vi "popUPCrearNuevoObjetoReceta.vi"() -> (2 "datosReceta":T1, 3 "Listo Ingresar OD SteelGrade Lote":bool=TRUE)   [LabVIEW 2014]
panel:
  in  "textoFinCarga":string="Gracias por ingresar los datos de la receta"
  in  "ingresarIDStadisctic":string="numeroIdStad"
  in  "ingresarDataCreate":string="camposMedicion"
  in  "ingresarIDReceta":string="numeroIDReceta"
  in  "ingresarCamposMedicion":string="numLote"
  in  "ingresarSteelGrade":string="numSteelGrade"
  in  "ingresarOD":string="numeroOD"
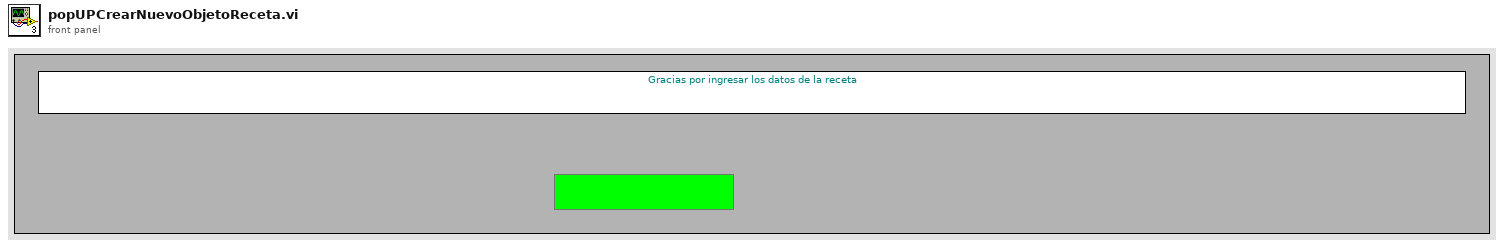
[diagram p1: front panel]
types:
  T1 = cluster{"idReceta":string, "od":string, "sg":string, "camposMedicion":string, "dataCreate":string, "idStadistic":string}
  T2 = enum8{"Enabled", "Disabled", "Disabled and Grayed Out"}
  T3 = cluster{string, string, string, string, string, string}
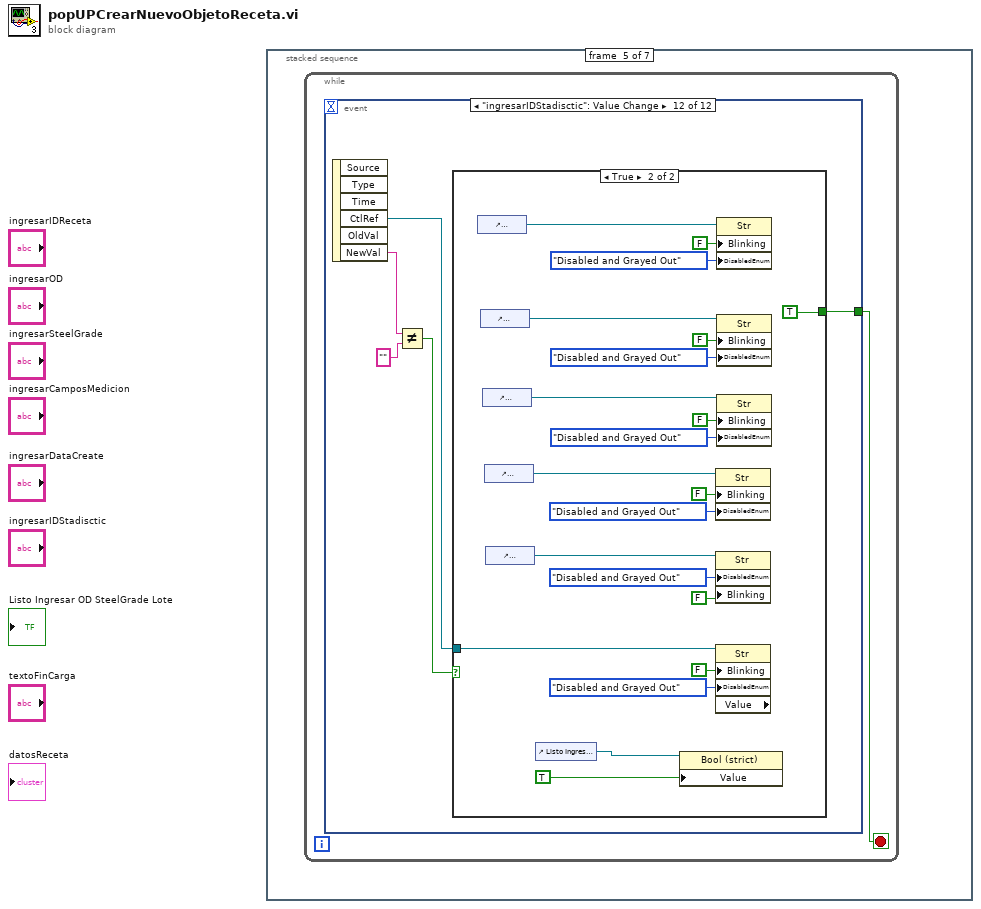
[diagram p0: block diagram]
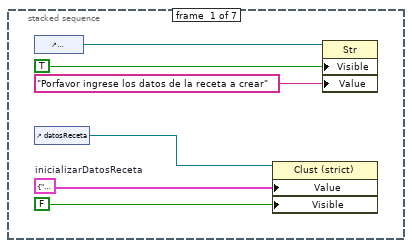
[diagram p2: hidden frame]
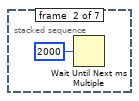
[diagram p3: hidden frame]
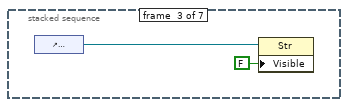
[diagram p4: hidden frame]
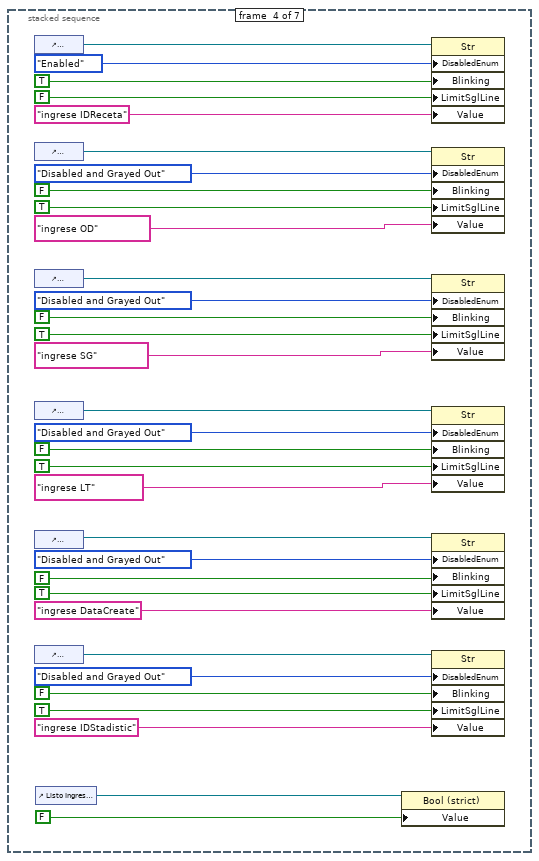
[diagram p5: hidden frame]
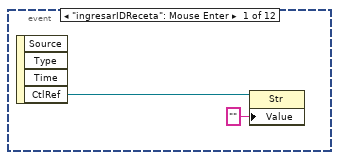
[diagram p6: hidden frame]
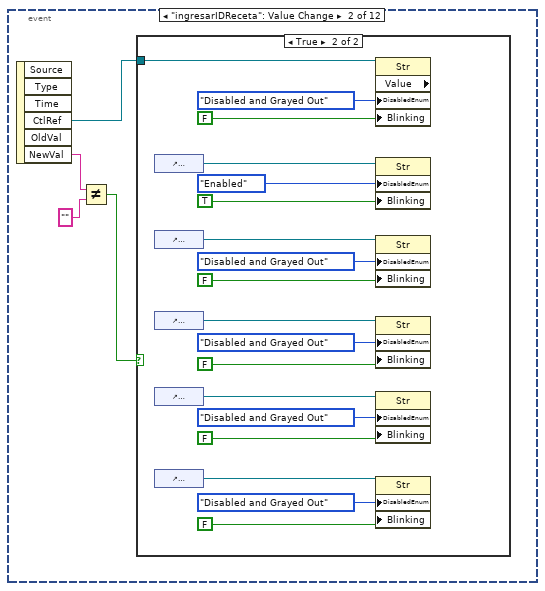
[diagram p7: hidden frame]
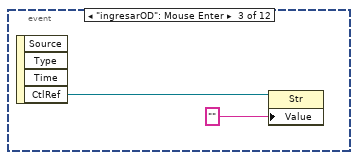
[diagram p9: hidden frame]
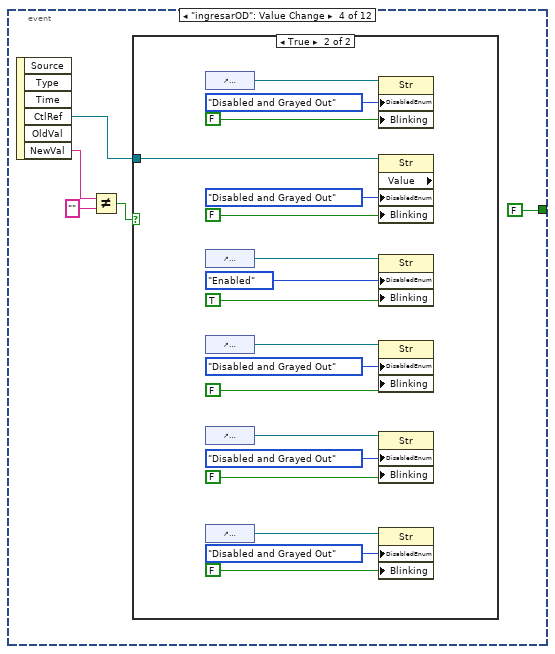
[diagram p10: hidden frame]
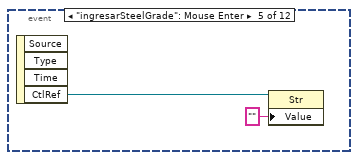
[diagram p12: hidden frame]
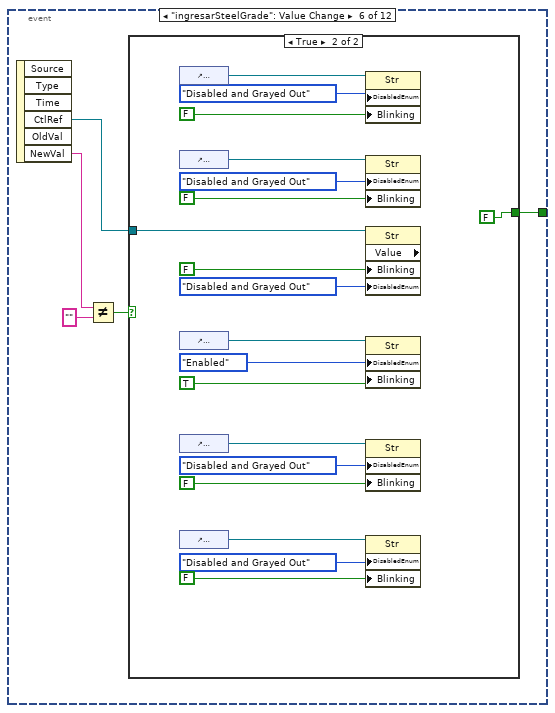
[diagram p13: hidden frame]
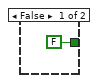
[diagram p14: hidden frame]
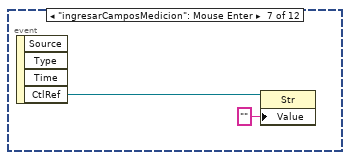
[diagram p15: hidden frame]
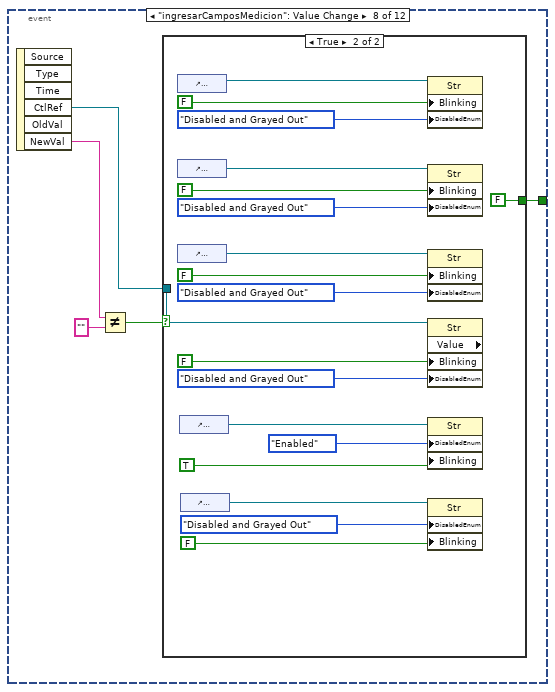
[diagram p16: hidden frame]
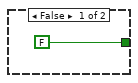
[diagram p17: hidden frame]
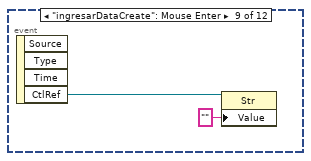
[diagram p18: hidden frame]
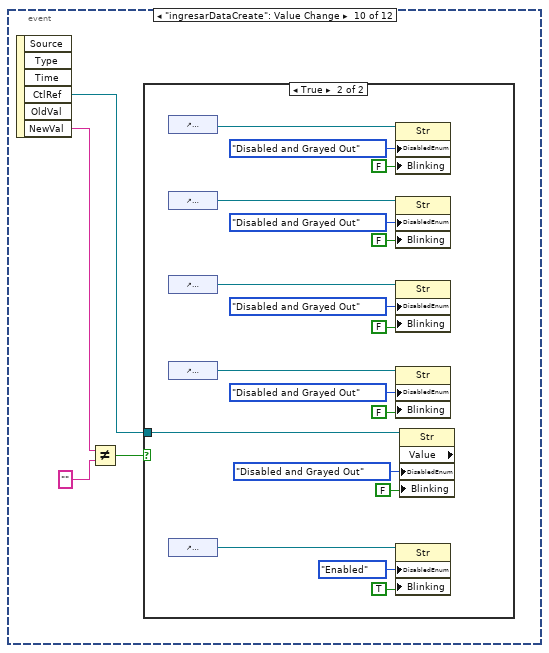
[diagram p19: hidden frame]
diagram:
  n1 = stacked-sequence {
    frame #0 {
      w1 = T3 {"", "", "", "", "", ""}  # inicializarDatosReceta
      n2 = control-ref of="textoFinCarga"() -> (w6:refnum<vi>)
      n3 = control-ref of="datosReceta"() -> (w2:refnum<vi>)
      n4 = property class="Clust (strict)"(reference=w2, "Value"=w1, "Visible"=FALSE) -> ()  [unwired: 1 in, 2 out]
      n5 = property class="Str"(reference=w6, "Visible"=TRUE, "Value"="Porfavor ingrese los datos de la receta a crear") -> ()  [unwired: 1 in, 2 out]
    }
    frame #1 {
      n6 = Wait Until Next ms Multiple(millisecond multiple=u32 2000) -> ()  [unwired: 1 out]
    }
    frame #2 {
      n7 = control-ref of="textoFinCarga"() -> (w9:refnum<vi>)
      n8 = property class="Str"(reference=w9, "Visible"=FALSE) -> ()  [unwired: 1 in, 2 out]
    }
    frame #3 {
      n9 = control-ref of="ingresarIDReceta"() -> (w24:refnum<vi>)
      n10 = control-ref of="ingresarOD"() -> (w41:refnum<vi>)
      n11 = control-ref of="ingresarSteelGrade"() -> (w39:refnum<vi>)
      n12 = control-ref of="ingresarCamposMedicion"() -> (w37:refnum<vi>)
      n13 = control-ref of="ingresarDataCreate"() -> (w19:refnum<vi>)
      n14 = control-ref of="ingresarIDStadisctic"() -> (w14:refnum<vi>)
      n15 = control-ref of="Listo Ingresar OD SteelGrade Lote"() -> (w29:refnum<vi>)
      n16 = property class="Bool (strict)"(reference=w29, "Value"=FALSE) -> ()  [unwired: 1 in, 2 out]
      n17 = property class="Str"(reference=w24, "DisabledEnum"=T2."Enabled" ("Disabled"), "Blinking"=TRUE, "LimitSglLine"=FALSE ("Limit To Single Line?"), "Value"="ingrese IDReceta") -> ()  [unwired: 1 in, 2 out]
      n18 = property class="Str"(reference=w41, "DisabledEnum"=T2."Disabled and Grayed Out" ("Disabled"), "Blinking"=FALSE, "LimitSglLine"=TRUE ("Limit To Single Line?"), "Value"="ingrese OD") -> ()  [unwired: 1 in, 2 out]
      n19 = property class="Str"(reference=w39, "DisabledEnum"=T2."Disabled and Grayed Out" ("Disabled"), "Blinking"=FALSE, "LimitSglLine"=TRUE ("Limit To Single Line?"), "Value"="ingrese SG") -> ()  [unwired: 1 in, 2 out]
      n20 = property class="Str"(reference=w37, "DisabledEnum"=T2."Disabled and Grayed Out" ("Disabled"), "Blinking"=FALSE, "LimitSglLine"=TRUE ("Limit To Single Line?"), "Value"="ingrese LT") -> ()  [unwired: 1 in, 2 out]
      n21 = property class="Str"(reference=w19, "DisabledEnum"=T2."Disabled and Grayed Out" ("Disabled"), "Blinking"=FALSE, "LimitSglLine"=TRUE ("Limit To Single Line?"), "Value"="ingrese DataCreate") -> ()  [unwired: 1 in, 2 out]
      n22 = property class="Str"(reference=w14, "DisabledEnum"=T2."Disabled and Grayed Out" ("Disabled"), "Blinking"=FALSE, "LimitSglLine"=TRUE ("Limit To Single Line?"), "Value"="ingrese IDStadistic") -> ()  [unwired: 1 in, 2 out]
    }
    frame #4 {
      n23 = while {
        stop <- w42 stop-if-true
        n24 = event shown="[11] \"ingresarIDStadisctic\": Value Change" {
          selector: _ -> [_ _ _ _ _ _ _ _ _ _ _ _]
          dyn-events: _ -> [_ _ _ _ _ _ _ _ _ _ _ _]
          timeout: _ -> [_ _ _ _ _ _ _ _ _ _ _ _]
          tunnel: [_ _ _ FALSE _ w97 _ w124 _ _ _ w172] -> w42
          event "ingresarIDReceta": Mouse Enter {
            n25 = event-data() -> ("CtlRef"=w44:refnum<vi>)  [unwired: 1 in, 3 out]
            n26 = property class="Str"(reference=w44, "Value"="") -> ()  [unwired: 1 in, 2 out]
          }
          event "ingresarIDReceta": Value Change {
            n27 = event-data() -> ("CtlRef"=w45:refnum<vi>, "NewVal"=w48:string)  [unwired: 1 in, 4 out]
            n28 = Not Equal?(x=w48, y="") -> (x != y?=w46:bool)
            n29 = case shown="True" w46 {
              tunnel: w45 -> [_ w66]
              frame False {
              }
              frame True {
                n30 = control-ref of="ingresarOD"() -> (w63:refnum<vi>)
                n31 = control-ref of="ingresarSteelGrade"() -> (w60:refnum<vi>)
                n32 = control-ref of="ingresarCamposMedicion"() -> (w57:refnum<vi>)
                n33 = control-ref of="ingresarDataCreate"() -> (w54:refnum<vi>)
                n34 = control-ref of="ingresarIDStadisctic"() -> (w51:refnum<vi>)
                n35 = property class="Str" props=["Value", "DisabledEnum", "Blinking"](reference=w66, "DisabledEnum"=T2."Disabled and Grayed Out" ("Disabled"), "Blinking"=FALSE) -> ()  [unwired: 1 in, 3 out]
                n36 = property class="Str"(reference=w63, "DisabledEnum"=T2."Enabled" ("Disabled"), "Blinking"=TRUE) -> ()  [unwired: 1 in, 2 out]
                n37 = property class="Str"(reference=w60, "DisabledEnum"=T2."Disabled and Grayed Out" ("Disabled"), "Blinking"=FALSE) -> ()  [unwired: 1 in, 2 out]
                n38 = property class="Str"(reference=w57, "DisabledEnum"=T2."Disabled and Grayed Out" ("Disabled"), "Blinking"=FALSE) -> ()  [unwired: 1 in, 2 out]
                n39 = property class="Str"(reference=w54, "DisabledEnum"=T2."Disabled and Grayed Out" ("Disabled"), "Blinking"=FALSE) -> ()  [unwired: 1 in, 2 out]
                n40 = property class="Str"(reference=w51, "DisabledEnum"=T2."Disabled and Grayed Out" ("Disabled"), "Blinking"=FALSE) -> ()  [unwired: 1 in, 2 out]
              }
            }
          }
          event "ingresarOD": Mouse Enter {
            n41 = event-data() -> ("CtlRef"=w68:refnum<vi>)  [unwired: 1 in, 3 out]
            n42 = property class="Str"(reference=w68, "Value"="") -> ()  [unwired: 1 in, 2 out]
          }
          event "ingresarOD": Value Change {
            n43 = event-data() -> ("CtlRef"=w73:refnum<vi>, "NewVal"=w69:string)  [unwired: 1 in, 4 out]
            n44 = Not Equal?(x=w69, y="") -> (x != y?=w71:bool)
            n45 = case shown="True" w71 {
              tunnel: w73 -> [_ w91]
              frame False {
              }
              frame True {
                n46 = control-ref of="ingresarIDReceta"() -> (w82:refnum<vi>)
                n47 = control-ref of="ingresarSteelGrade"() -> (w88:refnum<vi>)
                n48 = control-ref of="ingresarCamposMedicion"() -> (w85:refnum<vi>)
                n49 = control-ref of="ingresarDataCreate"() -> (w79:refnum<vi>)
                n50 = control-ref of="ingresarIDStadisctic"() -> (w76:refnum<vi>)
                n51 = property class="Str"(reference=w82, "DisabledEnum"=T2."Disabled and Grayed Out" ("Disabled"), "Blinking"=FALSE) -> ()  [unwired: 1 in, 2 out]
                n52 = property class="Str" props=["Value", "DisabledEnum", "Blinking"](reference=w91, "DisabledEnum"=T2."Disabled and Grayed Out" ("Disabled"), "Blinking"=FALSE) -> ()  [unwired: 1 in, 3 out]
                n53 = property class="Str"(reference=w88, "DisabledEnum"=T2."Enabled" ("Disabled"), "Blinking"=TRUE) -> ()  [unwired: 1 in, 2 out]
                n54 = property class="Str"(reference=w85, "DisabledEnum"=T2."Disabled and Grayed Out" ("Disabled"), "Blinking"=FALSE) -> ()  [unwired: 1 in, 2 out]
                n55 = property class="Str"(reference=w79, "DisabledEnum"=T2."Disabled and Grayed Out" ("Disabled"), "Blinking"=FALSE) -> ()  [unwired: 1 in, 2 out]
                n56 = property class="Str"(reference=w76, "DisabledEnum"=T2."Disabled and Grayed Out" ("Disabled"), "Blinking"=FALSE) -> ()  [unwired: 1 in, 2 out]
              }
            }
          }
          event "ingresarSteelGrade": Mouse Enter {
            n57 = event-data() -> ("CtlRef"=w93:refnum<vi>)  [unwired: 1 in, 3 out]
            n58 = property class="Str"(reference=w93, "Value"="") -> ()  [unwired: 1 in, 2 out]
          }
          event "ingresarSteelGrade": Value Change {
            n59 = event-data() -> ("CtlRef"=w98:refnum<vi>, "NewVal"=w96:string)  [unwired: 1 in, 4 out]
            n60 = Not Equal?(x=w96, y="") -> (x != y?=w94:bool)
            n61 = case shown="True" w94 {
              tunnel: w98 -> [_ w118]
              tunnel: [FALSE FALSE] -> w97
              frame False {
              }
              frame True {
                n62 = control-ref of="ingresarIDReceta"() -> (w111:refnum<vi>)
                n63 = control-ref of="ingresarOD"() -> (w110:refnum<vi>)
                n64 = control-ref of="ingresarCamposMedicion"() -> (w116:refnum<vi>)
                n65 = control-ref of="ingresarDataCreate"() -> (w105:refnum<vi>)
                n66 = control-ref of="ingresarIDStadisctic"() -> (w102:refnum<vi>)
                n67 = property class="Str"(reference=w111, "DisabledEnum"=T2."Disabled and Grayed Out" ("Disabled"), "Blinking"=FALSE) -> ()  [unwired: 1 in, 2 out]
                n68 = property class="Str"(reference=w110, "DisabledEnum"=T2."Disabled and Grayed Out" ("Disabled"), "Blinking"=FALSE) -> ()  [unwired: 1 in, 2 out]
                n69 = property class="Str" props=["Value", "Blinking", "DisabledEnum"](reference=w118, "Blinking"=FALSE, "DisabledEnum"=T2."Disabled and Grayed Out" ("Disabled")) -> ()  [unwired: 1 in, 3 out]
                n70 = property class="Str"(reference=w116, "DisabledEnum"=T2."Enabled" ("Disabled"), "Blinking"=TRUE) -> ()  [unwired: 1 in, 2 out]
                n71 = property class="Str"(reference=w105, "DisabledEnum"=T2."Disabled and Grayed Out" ("Disabled"), "Blinking"=FALSE) -> ()  [unwired: 1 in, 2 out]
                n72 = property class="Str"(reference=w102, "DisabledEnum"=T2."Disabled and Grayed Out" ("Disabled"), "Blinking"=FALSE) -> ()  [unwired: 1 in, 2 out]
              }
            }
          }
          event "ingresarCamposMedicion": Mouse Enter {
            n73 = event-data() -> ("CtlRef"=w120:refnum<vi>)  [unwired: 1 in, 3 out]
            n74 = property class="Str"(reference=w120, "Value"="") -> ()  [unwired: 1 in, 2 out]
          }
          event "ingresarCamposMedicion": Value Change {
            n75 = event-data() -> ("CtlRef"=w125:refnum<vi>, "NewVal"=w123:string)  [unwired: 1 in, 4 out]
            n76 = Not Equal?(x=w123, y="") -> (x != y?=w122:bool)
            n77 = case shown="True" w122 {
              tunnel: w125 -> [_ w145]
              tunnel: [FALSE FALSE] -> w124
              frame False {
              }
              frame True {
                n78 = control-ref of="ingresarIDReceta"() -> (w135:refnum<vi>)
                n79 = control-ref of="ingresarOD"() -> (w141:refnum<vi>)
                n80 = control-ref of="ingresarSteelGrade"() -> (w138:refnum<vi>)
                n81 = control-ref of="ingresarDataCreate"() -> (w132:refnum<vi>)
                n82 = control-ref of="ingresarIDStadisctic"() -> (w129:refnum<vi>)
                n83 = property class="Str"(reference=w135, "Blinking"=FALSE, "DisabledEnum"=T2."Disabled and Grayed Out" ("Disabled")) -> ()  [unwired: 1 in, 2 out]
                n84 = property class="Str"(reference=w141, "Blinking"=FALSE, "DisabledEnum"=T2."Disabled and Grayed Out" ("Disabled")) -> ()  [unwired: 1 in, 2 out]
                n85 = property class="Str"(reference=w138, "Blinking"=FALSE, "DisabledEnum"=T2."Disabled and Grayed Out" ("Disabled")) -> ()  [unwired: 1 in, 2 out]
                n86 = property class="Str" props=["Value", "Blinking", "DisabledEnum"](reference=w145, "Blinking"=FALSE, "DisabledEnum"=T2."Disabled and Grayed Out" ("Disabled")) -> ()  [unwired: 1 in, 3 out]
                n87 = property class="Str"(reference=w132, "DisabledEnum"=T2."Enabled" ("Disabled"), "Blinking"=TRUE) -> ()  [unwired: 1 in, 2 out]
                n88 = property class="Str"(reference=w129, "DisabledEnum"=T2."Disabled and Grayed Out" ("Disabled"), "Blinking"=FALSE) -> ()  [unwired: 1 in, 2 out]
              }
            }
          }
          event "ingresarDataCreate": Mouse Enter {
            n89 = event-data() -> ("CtlRef"=w147:refnum<vi>)  [unwired: 1 in, 3 out]
            n90 = property class="Str"(reference=w147, "Value"="") -> ()  [unwired: 1 in, 2 out]
          }
          event "ingresarDataCreate": Value Change {
            n91 = event-data() -> ("CtlRef"=w148:refnum<vi>, "NewVal"=w151:string)  [unwired: 1 in, 4 out]
            n92 = Not Equal?(x=w151, y="") -> (x != y?=w149:bool)
            n93 = case shown="True" w149 {
              tunnel: w148 -> [_ w169]
              frame False {
              }
              frame True {
                n94 = control-ref of="ingresarIDReceta"() -> (w168:refnum<vi>)
                n95 = control-ref of="ingresarOD"() -> (w167:refnum<vi>)
                n96 = control-ref of="ingresarSteelGrade"() -> (w166:refnum<vi>)
                n97 = control-ref of="ingresarCamposMedicion"() -> (w165:refnum<vi>)
                n98 = control-ref of="ingresarIDStadisctic"() -> (w164:refnum<vi>)
                n99 = property class="Str"(reference=w168, "DisabledEnum"=T2."Disabled and Grayed Out" ("Disabled"), "Blinking"=FALSE) -> ()  [unwired: 1 in, 2 out]
                n100 = property class="Str"(reference=w167, "DisabledEnum"=T2."Disabled and Grayed Out" ("Disabled"), "Blinking"=FALSE) -> ()  [unwired: 1 in, 2 out]
                n101 = property class="Str"(reference=w166, "DisabledEnum"=T2."Disabled and Grayed Out" ("Disabled"), "Blinking"=FALSE) -> ()  [unwired: 1 in, 2 out]
                n102 = property class="Str"(reference=w165, "DisabledEnum"=T2."Disabled and Grayed Out" ("Disabled"), "Blinking"=FALSE) -> ()  [unwired: 1 in, 2 out]
                n103 = property class="Str"(reference=w164, "DisabledEnum"=T2."Enabled" ("Disabled"), "Blinking"=TRUE) -> ()  [unwired: 1 in, 2 out]
                n104 = property class="Str" props=["Value", "DisabledEnum", "Blinking"](reference=w169, "DisabledEnum"=T2."Disabled and Grayed Out" ("Disabled"), "Blinking"=FALSE) -> ()  [unwired: 1 in, 3 out]
              }
            }
          }
          event "ingresarIDStadisctic": Mouse Enter {
            n105 = event-data() -> ("CtlRef"=w171:refnum<vi>)  [unwired: 1 in, 3 out]
            n106 = property class="Str"(reference=w171, "Value"="") -> ()  [unwired: 1 in, 2 out]
          }
          event "ingresarIDStadisctic": Value Change {
            n107 = event-data() -> ("CtlRef"=w173:refnum<vi>, "NewVal"=w176:string)  [unwired: 1 in, 4 out]
            n108 = Not Equal?(x=w176, y="") -> (x != y?=w174:bool)
            n109 = case shown="True" w174 {
              tunnel: w173 -> [_ w193]
              tunnel: [FALSE TRUE] -> w172
              frame False {
              }
              frame True {
                n110 = control-ref of="ingresarIDReceta"() -> (w198:refnum<vi>)
                n111 = control-ref of="ingresarOD"() -> (w197:refnum<vi>)
                n112 = control-ref of="ingresarSteelGrade"() -> (w196:refnum<vi>)
                n113 = control-ref of="ingresarCamposMedicion"() -> (w195:refnum<vi>)
                n114 = control-ref of="ingresarDataCreate"() -> (w194:refnum<vi>)
                n115 = control-ref of="Listo Ingresar OD SteelGrade Lote"() -> (w179:refnum<vi>)
                n116 = property class="Bool (strict)"(reference=w179, "Value"=TRUE) -> ()  [unwired: 1 in, 2 out]
                n117 = property class="Str"(reference=w195, "Blinking"=FALSE, "DisabledEnum"=T2."Disabled and Grayed Out" ("Disabled")) -> ()  [unwired: 1 in, 2 out]
                n118 = property class="Str"(reference=w194, "DisabledEnum"=T2."Disabled and Grayed Out" ("Disabled"), "Blinking"=FALSE) -> ()  [unwired: 1 in, 2 out]
                n119 = property class="Str" props=["Blinking", "DisabledEnum", "Value"](reference=w193, "Blinking"=FALSE, "DisabledEnum"=T2."Disabled and Grayed Out" ("Disabled")) -> ()  [unwired: 1 in, 3 out]
                n120 = property class="Str"(reference=w198, "Blinking"=FALSE, "DisabledEnum"=T2."Disabled and Grayed Out" ("Disabled")) -> ()  [unwired: 1 in, 2 out]
                n121 = property class="Str"(reference=w197, "Blinking"=FALSE, "DisabledEnum"=T2."Disabled and Grayed Out" ("Disabled")) -> ()  [unwired: 1 in, 2 out]
                n122 = property class="Str"(reference=w196, "Blinking"=FALSE, "DisabledEnum"=T2."Disabled and Grayed Out" ("Disabled")) -> ()  [unwired: 1 in, 2 out]
              }
            }
          }
        }
      }
    }
    frame #5 {
      n123 = control-ref of="textoFinCarga"() -> (w201:refnum<vi>)
      n124 = property class="Str"(reference=w201, "Value"="Gracias por ingresar los datos de la receta", "Visible"=TRUE) -> ()  [unwired: 1 in, 2 out]
    }
    frame #6 {
      w211 = T3 {"", "", "", "", "", ""}  # inicializarDatosReceta
      n125 = control-ref of="ingresarIDStadisctic"() -> (w208:refnum<vi>)
      n126 = control-ref of="ingresarDataCreate"() -> (w209:refnum<vi>)
      n127 = control-ref of="ingresarOD"() -> (w216:refnum<vi>)
      n128 = control-ref of="ingresarSteelGrade"() -> (w215:refnum<vi>)
      n129 = control-ref of="ingresarCamposMedicion"() -> (w214:refnum<vi>)
      n130 = control-ref of="ingresarIDReceta"() -> (w210:refnum<vi>)
      n131 = property class="Str"(reference=w210) -> ("Value"=w202:string)  [unwired: 1 in, 2 out]
      n132 = property class="Str"(reference=w216) -> ("Value"=w203:string)  [unwired: 1 in, 2 out]
      n133 = property class="Str"(reference=w215) -> ("Value"=w204:string)  [unwired: 1 in, 2 out]
      n134 = property class="Str"(reference=w209) -> ("Value"=w206:string)  [unwired: 1 in, 2 out]
      n135 = property class="Str"(reference=w208) -> ("Value"=w207:string)  [unwired: 1 in, 2 out]
      n136 = property class="Str"(reference=w214) -> ("Value"=w205:string)  [unwired: 1 in, 2 out]
      n137 = Wait Until Next ms Multiple(millisecond multiple=u32 2000) -> ()  [unwired: 1 out]
      n138 = Bundle(cluster=w211, w202, w203, w204, w205, w206, w207) -> (w213:T3)
      n139 = control-ref of="datosReceta"() -> (w212:refnum<vi>)
      n140 = property class="Clust (strict)"(reference=w212, "Value"=w213) -> ()  [unwired: 1 in, 2 out]
    }
  }
